vi "Save As Raw.vi"(10 "typ":i32, 11 "szFileTitle":string) -> (2 "function return":u32, 3 "szFileTitle out":string)   [LabVIEW 2018, in "Copy of Andor SDK.lvlib"]
doc: "EXPNETTYPE unsigned int WINAPI SaveAsRaw(char * szFileTitle, int typ);"
uses:
  Copy of Andor SDK.lvlib
  <userlib>/Andor SDK/ATMCD32D.dll
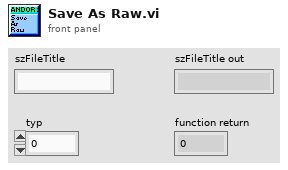
[diagram p1: front panel]
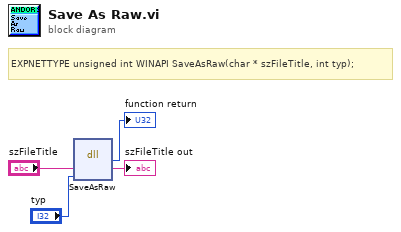
[diagram p0: block diagram]
diagram:
  # "EXPNETTYPE unsigned int WINAPI SaveAsRaw(char * szFileTitle, int typ);"
  n1 = dll-call lib="C:/Program Files (x86)/National Instruments/LabVIEW 2018/user.lib/Andor SDK/ATMCD32D.*" fn="SaveAsRaw"("szFileTitle"="szFileTitle", "typ"="typ") -> (→"function return":u32, "szFileTitle"=→"szFileTitle out":string)  [unwired: 4 in, 2 out]
